vi "12.2-6 ConvexHull.vi"() -> ()   [LabVIEW 2016]
doc: "This example shows how to use the Edge Tool in NI Vision. The Edge Tool finds edges (or sharp transitions in the pixels values) along a given line or ROI profile. The Edge Tool is a precursor function to many of the gauging and inspection tasks. For example, the location of the edges found along a line profile across an object can interpreted as the boundaries of the object whose dimensions have to be measured for a gauging application or the presence of a crack in the surface of an object for an inspection application."
uses:
  <vilib>/vision/NI_Vision_Development_Module.lvlib
panel:
  in  "Tab":T1(tab)
  out "Src":T2(plugin-control)
  out "Bin":T2(plugin-control)
  out "Dst":T2(plugin-control)
  in  "Range":cluster{"Lower value":sgl, "Upper value":sgl}={"Lower value"=0.0, "Upper value"=193.0}
  in  "Connectivity":bool=TRUE
  in  "Stop":bool
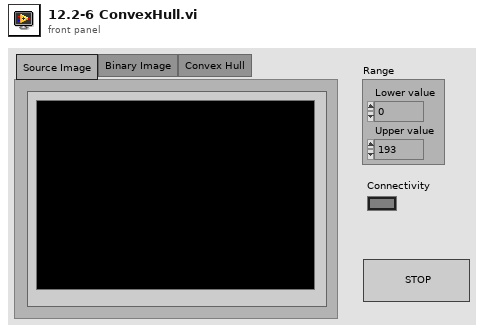
[diagram p1: front panel]
types:
  T1 = enum32{"Source Image", "Binary Image", "Convex Hull"}
  T2 = typedef "IMAQ Image.ctl" = refnum<image>
  T3 = cluster{"Range":cluster{"Lower value":sgl, "Upper value":sgl}, "Connectivity":bool}
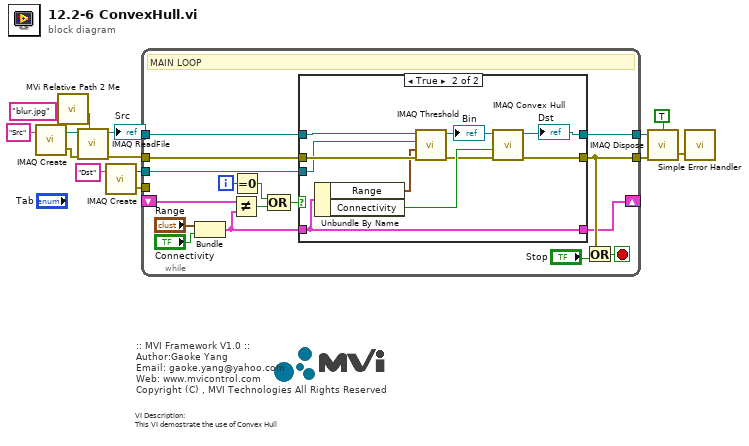
[diagram p0: block diagram]
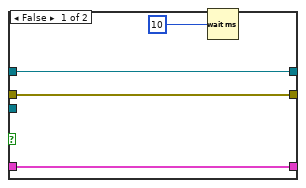
[diagram p2: hidden frame]
diagram:
  # "VI Description:\nThis VI demostrate the use of Convex Hull"
  # ":: MVI Framework V1.0 ::\nAuthor:Gaoke Yang\nEmail: gaoke.yang@yahoo.com\nWeb: www.mvicontrol.com\nCopyright (C) , MVI Technologies All Rights Reserved"
  n1 = call "IMAQ Create"("Image Name"="Src") -> ("New Image"=w13:T2, "error out"=w12:errorcluster)  [unwired: 4 in]
  n2 = call "MVi Relative Path 2 Me.vi"("Relative Path"="blur.jpg" ("name or relative path")) -> ("Appended Dir"=w8:path)  [unwired: 5 in, 1 out]
  n3 = call "IMAQ ReadFile"("File Path"=w8, "error in (no error)"=w12, "Image"=w13) -> ("error out"=w2:errorcluster, "Image Out"=w1:T2)  [unwired: 4 in, 3 out]
  "Src" <- w1
  n4 = call "IMAQ Create"("Image Name"="Dst") -> ("New Image"=w5:T2, "error out"=w4:errorcluster)  [unwired: 4 in]
  n5 = while "MAIN LOOP" {
    tunnel: w1 -> [w29]
    tunnel: w2 -> [w30]
    tunnel: [w25] -> w11
    tunnel: [w26] -> w10
    shift-right: [w22] -> _
    shift-left: _ -> [w20]
    tunnel: w5 -> [w18]
    tunnel: w4 -> [_]
    i -> [w24]
    stop <- w27 stop-if-true
    # "MAIN LOOP"
    n6 = Bundle("Range"="Range", "Connectivity"="Connectivity") -> (w15:T3)  [unwired: 1 in]
    n7 = Not Equal?(x=w20, y=w15) -> (x != y?=w19:bool)
    n8 = Equal To 0?(x=w24) -> (x = 0?=w21:bool)
    n9 = Compound Arithmetic op=OR(w21, w19) -> (w23:bool)
    n10 = case shown="True" w23 {
      tunnel: w30 -> [w33 w42]
      tunnel: w29 -> [w34 w41]
      tunnel: [w34 w43] -> w26
      tunnel: [w33 w44] -> w25
      tunnel: [w31 w40] -> w22
      tunnel: w15 -> [w31 w40]
      tunnel: w18 -> [_ w35]
      frame False {
        n11 = Wait (ms)(milliseconds to wait=u32 10) -> ()  [unwired: 1 out]
      }
      frame True {
        n12 = Unbundle By Name(w40) -> ("Range"=w39:cluster{"Lower value":sgl, "Upper value":sgl}, "Connectivity"=w38:bool)
        n13 = call "IMAQ Threshold"("error in (no error)"=w42, "Range"=w39, "Image Dst"=w35, "Image Src"=w41) -> ("error out"=w37:errorcluster, "Image Dst Out"=w36:T2)  [unwired: 6 in]
        "Bin" <- w36
        n14 = call "IMAQ Convex Hull"("error in (no error)"=w37, "Connectivity 4/8 (8)"=w38, "Image Src"=w36) -> ("error out"=w44:errorcluster, "Image Dst Out"=w43:T2)  [unwired: 7 in]
        "Dst" <- w43
      }
    }
    n15 = Or(x=w25, y="Stop") -> (x .or. y?=w27:bool)
  }
  n16 = call "IMAQ Dispose"("All Images? (No)"=TRUE, "Image"=w10, "error in (no error)"=w11) -> ("error out"=w7:errorcluster)  [unwired: 3 in]
  n17 = call <vilib>:"Simple Error Handler.vi"("error in (no error)"=w7) -> ()  [unwired: 4 in, 5 out]
